vi "CAN Get Value.vi"   [LabVIEW 2016]
doc: "Retrieves information from a PCAN Channel.\n\nParameters Description \nChannel The handle of a PCAN Channel (see TPCANHandle). \nParameter The code of the information to be retrieved. \nBuffer The buffer to return the required value. \nBufferLength The length in bytes of the given buffer. \n\nReturns:\nInputs and outputs of this Vi depend on the selected function.\nThe instances of the VI are in the Get Value path."
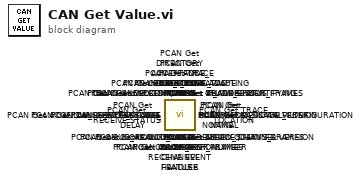
[diagram p0: block diagram]
diagram:
  n1 = call <instrlib>:"PCAN Get USB DEVICE NUMBER.vi"() -> ()  [unwired: 9 in, 3 out]
  n2 = call <instrlib>:"PCAN Get TRACE STATUS.vi"() -> ()  [unwired: 9 in, 3 out]
  n3 = call <instrlib>:"PCAN Get TRACE SIZE.vi"() -> ()  [unwired: 9 in, 3 out]
  n4 = call <instrlib>:"PCAN Get TRACE LOCATION.vi"() -> ()  [unwired: 9 in, 3 out]
  n5 = call <instrlib>:"PCAN Get TRACE CONFIGURE.vi"() -> ()  [unwired: 9 in, 3 out]
  n6 = call <instrlib>:"PCAN Get SPEED QUERY.vi"() -> ()  [unwired: 9 in, 3 out]
  n7 = call <instrlib>:"PCAN Get SPEED QUERY FD.vi"() -> ()  [unwired: 9 in, 3 out]
  n8 = call <instrlib>:"PCAN Get RECEIVE STATUS.vi"() -> ()  [unwired: 9 in, 3 out]
  n9 = call <instrlib>:"PCAN Get RECEIVE EVENT HANDLER .vi"() -> ()  [unwired: 9 in, 3 out]
  n10 = call <instrlib>:"PCAN Get MESSAGE FILTER.vi"() -> ()  [unwired: 9 in, 3 out]
  n11 = call <instrlib>:"PCAN Get LOG STATUS.vi"() -> ()  [unwired: 9 in, 3 out]
  n12 = call <instrlib>:"PCAN Get LOG LOCATION.vi"() -> ()  [unwired: 9 in, 3 out]
  n13 = call <instrlib>:"PCAN Get LOG CONFIGURE.vi"() -> ()  [unwired: 9 in, 3 out]
  n14 = call <instrlib>:"PCAN Get LISTEN ONLY.vi"() -> ()  [unwired: 9 in, 3 out]
  n15 = call <instrlib>:"PCAN Get LAN_SERVICE_STATUS.vi"() -> ()  [unwired: 10 in, 2 out]
  n16 = call <instrlib>:"PCAN Get IP_ADDRESS.vi"() -> ()  [unwired: 10 in, 2 out]
  n17 = call <instrlib>:"PCAN Get IO_DIGITAL_VALUE.vi"() -> ()  [unwired: 9 in, 3 out]
  n18 = call <instrlib>:"PCAN Get IO_DIGITAL_CONFIGURATION.vi"() -> ()  [unwired: 9 in, 3 out]
  n19 = call <instrlib>:"PCAN Get IO_ANALOG_VALUE.vi"() -> ()  [unwired: 9 in, 3 out]
  n20 = call <instrlib>:"PCAN Get INTERFRAME_DELAY  .vi"() -> ()  [unwired: 9 in, 3 out]
  n21 = call <instrlib>:"PCAN Get HARDWARE NAME.vi"() -> ()  [unwired: 9 in, 3 out]
  n22 = call <instrlib>:"PCAN Get DIRECTORY PATH FOR TRACE FILES.vi"() -> ()  [unwired: 10 in, 2 out]
  n23 = call <instrlib>:"PCAN Get DEVICE CHANNEL VERSION.vi"() -> ()  [unwired: 9 in, 3 out]
  n24 = call <instrlib>:"PCAN Get CONTROLLER NUMBER.vi"() -> ()  [unwired: 9 in, 3 out]
  n25 = call <instrlib>:"PCAN Get CHANNEL IDENTIFYING.vi"() -> ()  [unwired: 9 in, 3 out]
  n26 = call <instrlib>:"PCAN Get CHANNEL FEATURE.vi"() -> ()  [unwired: 9 in, 3 out]
  n27 = call <instrlib>:"PCAN Get CHANNEL CONDITION.vi"() -> ()  [unwired: 9 in, 3 out]
  n28 = call <instrlib>:"PCAN Get CAN BITRATE ADAPTING.vi"() -> ()  [unwired: 9 in, 3 out]
  n29 = call <instrlib>:"PCAN Get BUSSPEED_DATA.vi"() -> ()  [unwired: 9 in, 3 out]
  n30 = call <instrlib>:"PCAN Get BUSSPEED NOMINAL.vi"() -> ()  [unwired: 9 in, 3 out]
  n31 = call <instrlib>:"PCAN Get BUSOFF AUTORESET.vi"() -> ()  [unwired: 9 in, 3 out]
  n32 = call <instrlib>:"PCAN Get BASIC API VERSION.vi"() -> ()  [unwired: 10 in, 2 out]
  n33 = call <instrlib>:"PCAN Get ALLOW_STATUS_FRAMES.vi"() -> ()  [unwired: 9 in, 3 out]
  n34 = call <instrlib>:"PCAN Get ALLOW_RTR_FRAMES.vi"() -> ()  [unwired: 9 in, 3 out]
  n35 = call <instrlib>:"PCAN Get ALLOW_ERROR_FRAMES.vi"() -> ()  [unwired: 9 in, 3 out]
  n36 = call <instrlib>:"PCAN Get ACCEPTANCE_FILTER_29BIT.vi"() -> ()  [unwired: 9 in, 3 out]
  n37 = call <instrlib>:"PCAN Get ACCEPTANCE_FILTER_11BIT.vi"() -> ()  [unwired: 9 in, 3 out]
  n38 = call <instrlib>:"PCAN Get 5VOLTS POWER.vi"() -> ()  [unwired: 9 in, 3 out]
